vi "LMS on GIC 4.vi"(0 "GIC Input":T1={"Real/Sim"=FALSE, "WP Lats and Longs"={"WP Lats"=[], "WP Longs"=[]}, "GPS Time Int"=0.0, "GPS Com Port"="", "Compass Com Port"="", "Prop Com Port"="", "GPS Data"=[], "Compass"=0.0, "LMS Vector"=[], "Vision Vector"=[], "Direction Cmd"=0.0, "Speed Cmd"=0.0, "Time of Last GPS"=0.0, "WP Vector"=[], "WP Number"=0, "Num of WPs"=0, "SW Map"=[], "Obst Lats and Longs"={"Obst Lats"=[], "Obst Longs"=[]}, "Parameters"=[], "Path Cluster"={"Path x nodes"=[], "Path y nodes"=[]}, "     Use ?\nOff       On"=[TRUE, TRUE, FALSE, FALSE]} {"Obst Lats and Longs"."Obst Longs" format="%#_8g"; "Obst Lats and Longs"."Obst Lats" format="%#_8g"}, 5 "VISA resource name":refnum<visa-resource-name>, 9 "Numeric":i32) -> (4 "GIC Output":T1={"Real/Sim"=FALSE, "WP Lats and Longs"={"WP Lats"=[], "WP Longs"=[]}, "GPS Time Int"=0.0, "GPS Com Port"="", "Compass Com Port"="", "Prop Com Port"="", "GPS Data"=[], "Compass"=0.0, "LMS Vector"=[], "Vision Vector"=[], "Direction Cmd"=0.0, "Speed Cmd"=0.0, "Time of Last GPS"=0.0, "WP Vector"=[], "WP Number"=0, "Num of WPs"=0, "SW Map"=[], "Obst Lats and Longs"={"Obst Lats"=[], "Obst Longs"=[]}, "Parameters"=[], "Path Cluster"={"Path x nodes"=[], "Path y nodes"=[]}, "     Use ?\nOff       On"=[TRUE, TRUE, FALSE, FALSE]} {"Obst Lats and Longs"."Obst Longs" format="%#_8g"; "Obst Lats and Longs"."Obst Lats" format="%#_8g"})   [LabVIEW 2014]
uses:
  Hokuyo URG Series.lvlib
panel:
  out "Magnitude":dbl[](array[numeric])
  in  "Number of Scans":dbl
  in  "Scan Interval":dbl
  in  "Encoding Width":u16(ring)=3 items=["2 Byte"=2, "3 Byte"=3]
  in  "Cluster Count":dbl=1.0
  in  "Start Point":dbl=-135.0
  in  "End Point":dbl=135.0
  out "swmap":dbl[][](array[numeric])
  out "Boolean":bool
  out "lms vector":dbl[](array[numeric])
  # "LMS on GIC"
  # "GPS"
  # "LMS"
  # "Vision"
  # "Prop"
  # "GPS"
  # "LMS"
  # "Vision"
  # "Prop"
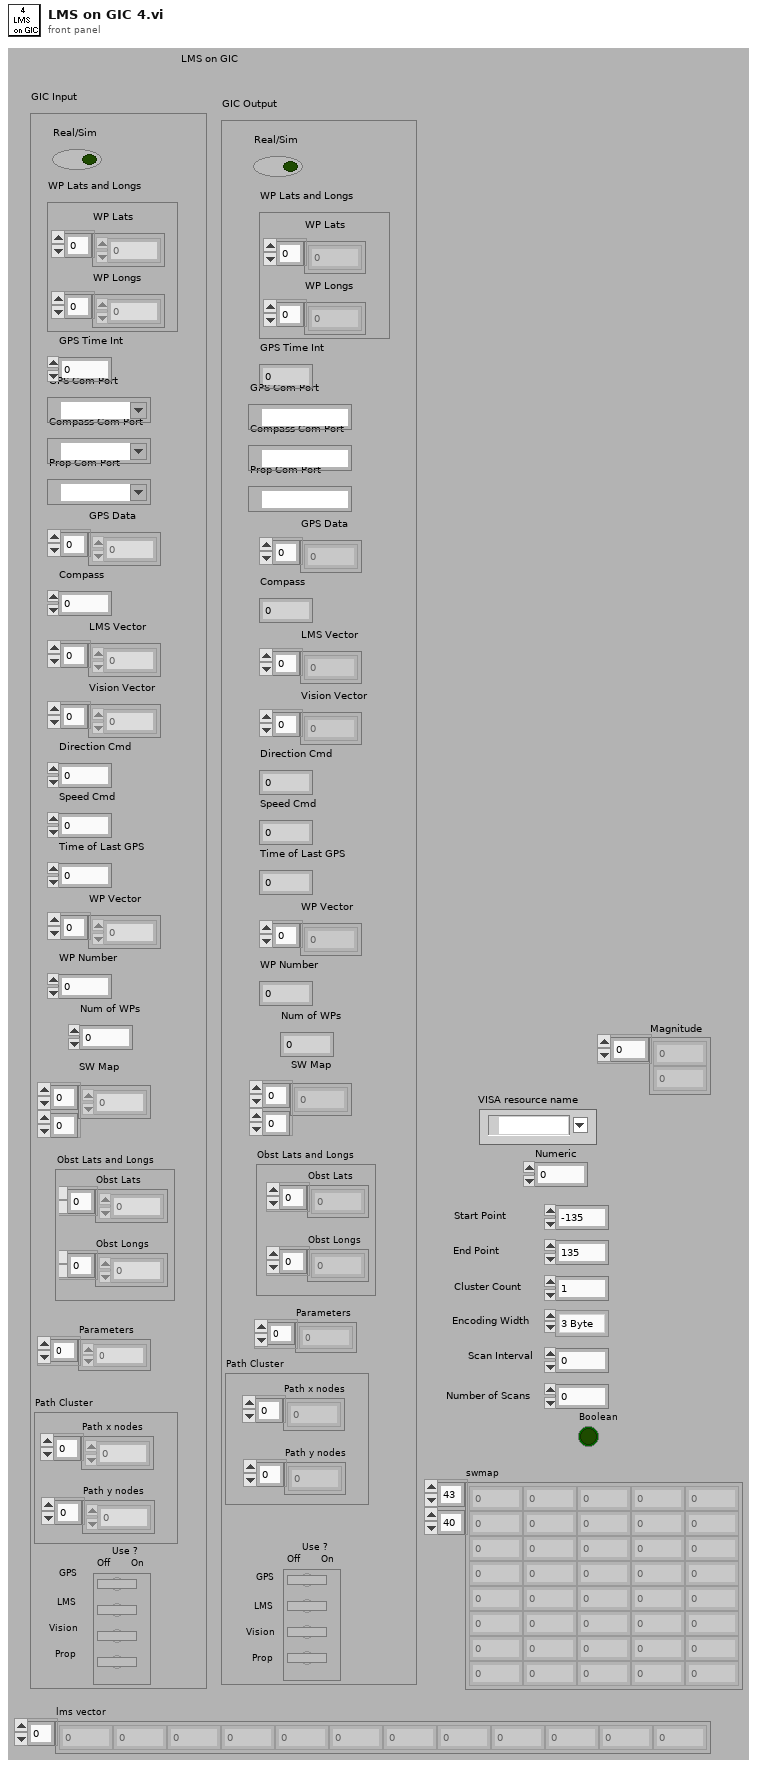
[diagram p1: front panel]
types:
  T1 = cluster{"Real/Sim":bool, "WP Lats and Longs":cluster{"WP Lats":dbl[], "WP Longs":dbl[]}, "GPS Time Int":dbl, "GPS Com Port":refnum<visa-resource-name>, "Compass Com Port":refnum<visa-resource-name>, "Prop Com Port":refnum<visa-resource-name>, "GPS Data":dbl[], "Compass":dbl, "LMS Vector":dbl[], "Vision Vector":dbl[], "Direction Cmd":dbl, "Speed Cmd":dbl, "Time of Last GPS":dbl, "WP Vector":dbl[], "WP Number":i32, "Num of WPs":i16, "SW Map":i32[][], "Obst Lats and Longs":cluster{"Obst Lats":dbl[], "Obst Longs":dbl[]}, "Parameters":dbl[], "Path Cluster":cluster{"Path x nodes":dbl[], "Path y nodes":dbl[]}, "     Use ?\nOff       On":bool[]}
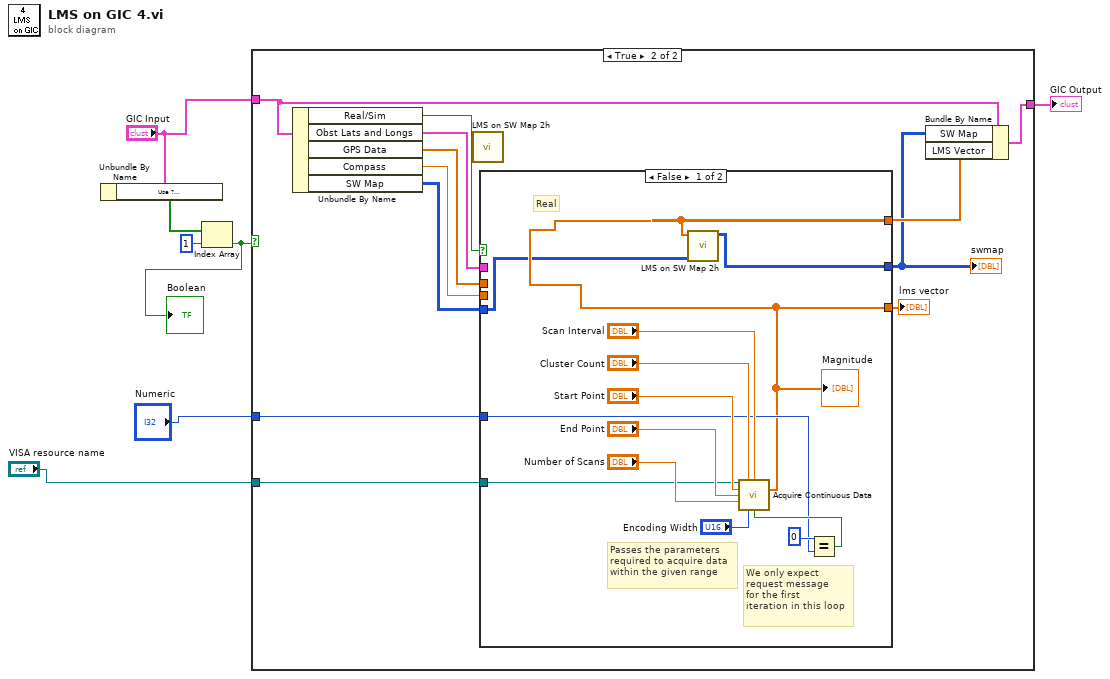
[diagram p0: block diagram]
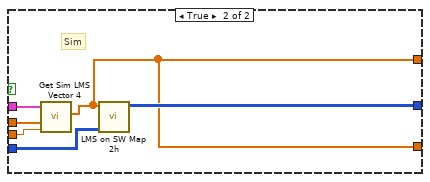
[diagram p3: hidden frame]
diagram:
  n1 = Unbundle By Name("GIC Input") -> ("Use ?\nOff       On"=w7:bool[])
  n2 = Index Array(array=w7, index=1) -> (element=w3:bool)
  "Boolean" <- w3
  n3 = case shown="True" w3 {
    tunnel: "GIC Input" -> [w8 w15]
    tunnel: [w8 w12] -> w4
    tunnel: "VISA resource name" -> [_ w11]
    tunnel: "Numeric" -> [_ w10]
    frame False {
    }
    frame True {
      n4 = Unbundle By Name(w15) -> ("Real/Sim"=w20:bool, "Obst Lats and Longs"=w19:cluster{"Obst Lats":dbl[], "Obst Longs":dbl[]}, "GPS Data"=w18:dbl[], "Compass"=w17:dbl, "SW Map"=w14:i32[][])
      n5 = call "LMS on SW Map 2h.vi"() -> ()  [unwired: 11 in, 1 out]
      n6 = case shown="False" w20 {
        tunnel: w19 -> [_ w38]
        tunnel: w18 -> [_ w39]
        tunnel: w17 -> [_ w37]
        tunnel: w14 -> [w22 w36]
        tunnel: [w21 w35] -> w9
        tunnel: [w23 w34] -> w16
        tunnel: [w23 w34] -> w13
        tunnel: w11 -> [w27 _]
        tunnel: w10 -> [w24 _]
        frame False {
          # "We only expect\nrequest message\nfor the first\niteration in this loop"
          # "Passes the parameters\nrequired to acquire data\nwithin the given range"
          # "Real"
          n7 = Equal?(x=0, y=w24) -> (x = y?=w25:bool)
          n8 = call "Acquire Continuous Data.vi"("VISA resource name"=w27, "Cluster Count (1)"="Cluster Count", "Scan Interval (1)"="Scan Interval", "Start Point (-120°)"="Start Point", "End Point (120°)"="End Point", "Number of Scans (0)"="Number of Scans", "Data Encoding Width (3 Byte)"="Encoding Width", "Enable Request Message (F:Disable)"=w25) -> ("Magnitude"=w23:dbl[])  [unwired: 2 in, 5 out]
          "Magnitude" <- w23
          n9 = call "LMS on SW Map 2h.vi"("SW Map In"=w22, "LMS Vector"=w23) -> ("SW Map Out"=w21:i32[][])  [unwired: 9 in]
        }
        frame True {
          # "Sim"
          n10 = call "Get Sim LMS Vector 4.vi"("Compass"=w37, "GPS Data"=w39, "Obst Lats and Longs"=w38) -> ("LMS Vector"=w34:dbl[])  [unwired: 8 in]
          n11 = call "LMS on SW Map 2h.vi"("SW Map In"=w36, "LMS Vector"=w34) -> ("SW Map Out"=w35:i32[][])  [unwired: 9 in]
        }
      }
      "lms vector" <- w13
      "swmap" <- w9
      n12 = Bundle By Name(cluster=w15, "SW Map"=w9, "LMS Vector"=w16) -> (w12:T1)
    }
  }
  "GIC Output" <- w4
